vi "setStateToState0.vi"(8 "error in (no error)":errorcluster, 11 "ZTAAC in":refnum<class "ZTAAC.lvclass">) -> (0 "error out":errorcluster, 3 "ZTAAC out":refnum<class "ZTAAC.lvclass">)   [LabVIEW 2016, in "OfcFunc.lvlib" / "ZTAAC.lvclass"]
doc: "Set the state to state 0."
uses:
  ZTAAC.lvclass
  ZTAAC.lvclass/ZTAAC.ctl
  OptCtrl/OptCtrl.lvclass
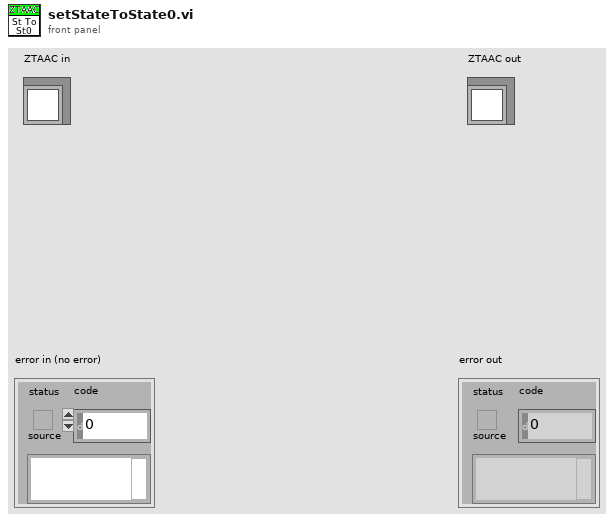
[diagram p1: front panel]
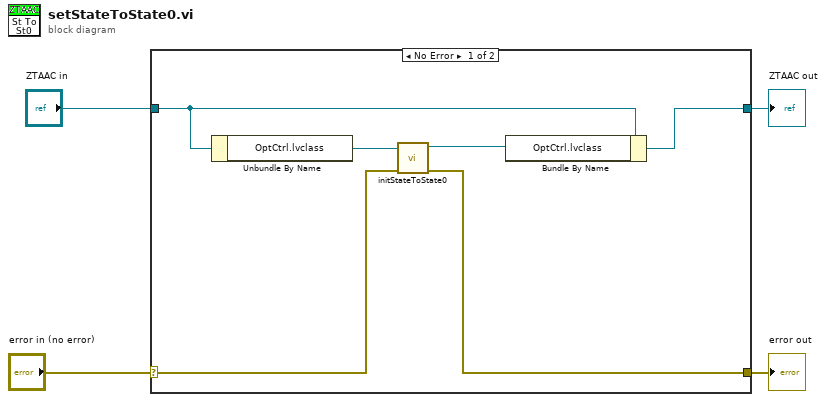
[diagram p0: block diagram]
diagram:
  n1 = case shown="No Error" "error in (no error)" {
    selector: "error in (no error)" -> [w9 w12]
    tunnel: [w8 w12] -> w3
    tunnel: [w5 w11] -> w1
    tunnel: "ZTAAC in" -> [w6 w11]
    frame No Error {
      n2 = Unbundle By Name(w6) -> ("OptCtrl.lvclass"=w10:refnum<class "OptCtrl.lvclass">)
      n3 = call "initStateToState0.vi"("error in (no error)"=w9, "OptCtrl in"=w10) -> ("error out"=w8:errorcluster, "OptCtrl out"=w7:refnum<class "OptCtrl.lvclass">)  [unwired: 8 in]
      n4 = Bundle By Name(cluster=w6, "OptCtrl.lvclass"=w7) -> (w5:refnum<class "ZTAAC.lvclass">)
    }
    frame Error {
    }
  }
  "error out" <- w3
  "ZTAAC out" <- w1
